vi "Read.vi"(8 "error in (no error)":errorcluster, 11 "Connection Handler in":refnum<class "Connection Handler.lvclass">) -> (0 "error out":errorcluster, 3 "Connection Handler out":refnum<class "Connection Handler.lvclass">)   [LabVIEW 2019, in "Network Interface.lvlib" / "Connection Handler.lvclass"]
uses:
  <vilib>/gpm_packages/@cs/Network-Sink/Source/Network Interface/Connection Handler/Connection Handler.lvclass
  <vilib>/gpm_packages/@cs/Network-Sink/Source/Network Interface/Connection Handler/Connection Handler.lvclass/Connection Handler.ctl
  <vilib>/gpm_packages/@cs/Network-Sink/Source/Network Interface/IMessagingProtocol/IMessagingProtocol.lvclass
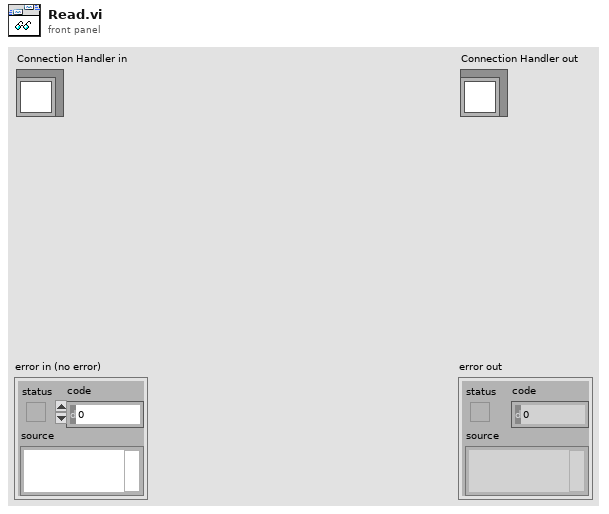
[diagram p1: front panel]
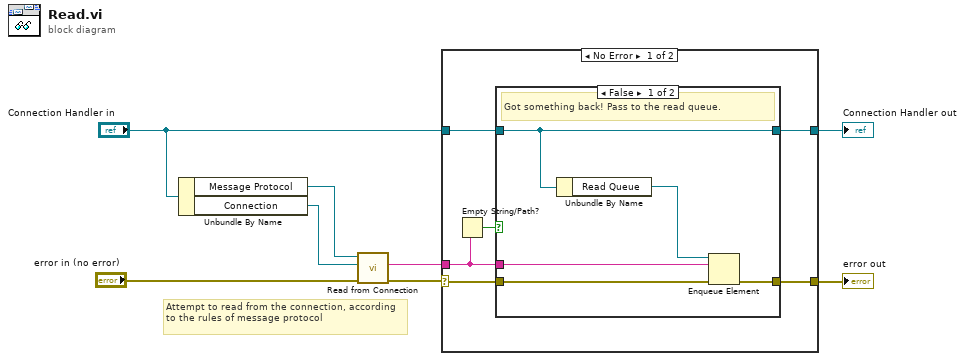
[diagram p0: block diagram]
diagram:
  # "Attempt to read from the connection, according to the rules of message protocol"
  n1 = Unbundle By Name("Connection Handler in") -> ("Message Protocol"=w7:refnum<class "IMessagingProtocol.lvclass">, "Connection"=w6:refnum<class "IConnection.lvclass">)
  n2 = call-dynamic "Read from Connection.vi"("error in (no error)"="error in (no error)", "Connection"=w6, "IMessagingProtocol in"=w7) -> ("error out"=w4:errorcluster, "Data Read"=w2:string)  [unwired: 6 in, 1 out]
  n3 = case shown="No Error" w4 {
    selector: w4 -> [w13 w23]
    tunnel: [w12 w23] -> w8
    tunnel: [w14 w22] -> w1
    tunnel: "Connection Handler in" -> [w9 w22]
    tunnel: w2 -> [w10 _]
    frame No Error {
      n4 = Empty String/Path?(string/path=w10) -> (empty?=w11:bool)
      n5 = case shown="False" w11 {
        tunnel: [w17 w20] -> w14
        tunnel: w13 -> [w16 w21]
        tunnel: [w15 w21] -> w12
        tunnel: w10 -> [w18 _]
        tunnel: w9 -> [w17 w20]
        frame False {
          # "Got something back! Pass to the read queue."
          n6 = Unbundle By Name(w17) -> ("Read Queue"=w19:refnum<queue>)
          n7 = Enqueue Element(queue=w19, element=w18, error in (no error)=w16) -> (error out=w15:errorcluster)  [unwired: 1 in, 2 out]
        }
        frame True {
          # "No data received"
        }
      }
    }
    frame Error {
    }
  }
  "error out" <- w8
  "Connection Handler out" <- w1
